vi "Wait Any.vi"(8 "error in (no error)":errorcluster, 9 "Timeout mS (-1)":i32=-1, 11 "Futures":refnum<class "Future.lvclass">[](array[class])) -> (0 "error out":errorcluster, 1 "Index":i32, 2 "Result":refnum<class>)   [LabVIEW 2020, in "Promises.lvlib" / "Future.lvclass"]
doc: "Waits for the first Result to be returned from several Futures and returns the index of the Future that provided the value. All specified Futures will become invalid after this VI."
uses:
  Future.lvclass
  Future.lvclass/Future.ctl
  Result State.ctl
  Promises.lvlib
  Result.ctl
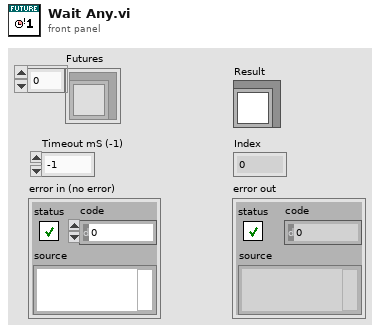
[diagram p1: front panel]
types:
  T1 = typedef "Promises.lvlib/Result.ctl" = cluster{"State":T2, "Value":refnum<class>}
  T2 = typedef "Promises.lvlib/Result State.ctl" = enum16{"Unset", "Error", "Success"}
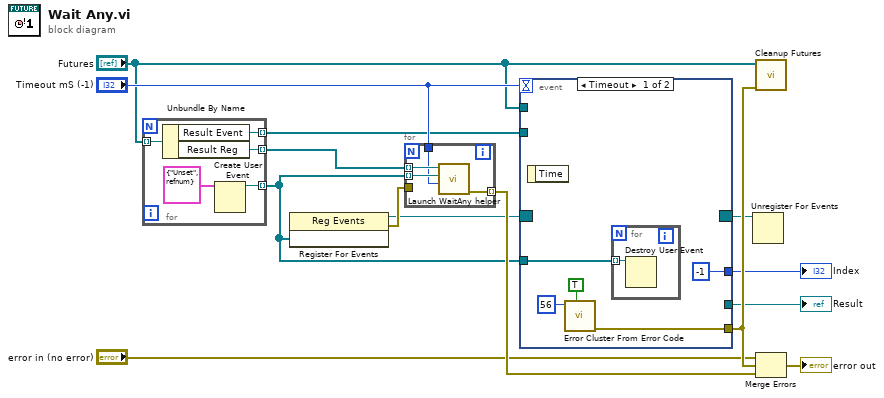
[diagram p0: block diagram]
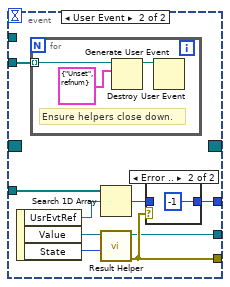
[diagram p2: hidden frame]
diagram:
  n1 = for {
    tunnel: "Futures" -> [w19] mode=indexing
    tunnel: [w17] -> w5 mode=indexing
    tunnel: [w16] -> w9 mode=indexing
    tunnel: [w15] -> w2 mode=indexing
    n2 = Unbundle By Name(w19) -> ("Result Event"=w15:refnum<user-event>, "Result Reg"=w16:refnum<event-registration>)
    n3 = Create User Event(user event datatype=T1 {"State"=enum."Unset", "Value"=refnum} ("Result")) -> (user event=w17:refnum<user-event>)  [unwired: 1 in, 1 out]
  }
  n4 = register-events(w5) -> (reference out=w10:refnum<event-registration>, error out=w12:errorcluster)  [unwired: 2 in]
  n5 = for {
    tunnel: w12 -> [_]
    tunnel: w9 -> [w23] mode=indexing
    tunnel: "Timeout mS (-1)" -> [w21]
    tunnel: w5 -> [w22] mode=indexing
    tunnel: [w20] -> w13 mode=indexing
    n6 = call "Launch WaitAny helper.vi"("Timeout"=w21, "Forwarded Event"=w22, "Event Reg"=w23) -> ("error out"=w20:errorcluster)  [unwired: 8 in]
  }
  n7 = event shown="[0] Timeout" {
    selector: w10 -> [_ _]
    dyn-events: [_ _] -> w6
    timeout: "Timeout mS (-1)" -> [_ _]
    tunnel: [_ w35] -> w4
    tunnel: [w28 w38] -> w14
    tunnel: w5 -> [w25 w34]
    tunnel: [-1 ("index of element") w31] -> w3
    tunnel: "Futures" -> [_ _]
    tunnel: w2 -> [_ w30]
    event Timeout {
      n8 = event-data() -> ()  [unwired: 1 in, 1 out]
      n9 = call <vilib>:"Error Cluster From Error Code.vi"("show call chain? (False)"=TRUE, "error code (0)"=56) -> ("error out"=w28:errorcluster)  [unwired: 7 in]
      n10 = for {
        tunnel: w25 -> [w29] mode=indexing
        n11 = Destroy User Event(user event=w29) -> ()  [unwired: 1 in, 1 out]
      }
    }
    event User Event {
      n12 = event-data() -> ("UsrEvtRef"=w33:refnum<user-event>, "Value"=w37:refnum<class>, "State"=w36:T2)  [unwired: 1 in]
      n13 = for {
        tunnel: w30 -> [w41] mode=indexing
        # "Ensure helpers close down."
        n14 = Generate User Event(user event=w41, event data cluster=T1 {"State"=enum."Unset", "Value"=refnum} ("event data")) -> (user event out=w39:refnum<user-event>)  [unwired: 2 in, 1 out]
        n15 = Destroy User Event(user event=w39) -> ()  [unwired: 1 in, 1 out]
      }
      n16 = Search 1D Array(1D array=w34, element=w33) -> (index of element=w32:i32)  [unwired: 1 in]
      n17 = call "Result Helper.vi"("State"=w36, "Value In"=w37) -> ("Error"=w38:errorcluster, "Value"=w35:refnum<class>)  [unwired: 8 in]
      n18 = case shown="Error .." w38 {
        tunnel: w32 -> [w42 _]
        tunnel: [w42 -1 ("index of element")] -> w31
        frame No Error {
        }
        frame Error {
        }
      }
    }
  }
  "Result" <- w4
  "Index" <- w3
  n19 = Unregister For Events(event registration refnum=w6) -> ()  [unwired: 1 in, 1 out]
  n20 = call "Cleanup Futures.vi"("error in (no error)"=w14, "Future in"="Futures") -> ()  [unwired: 10 in]
  n21 = Merge Errors("error in (no error)", w14, w13) -> (→"error out":errorcluster)
